vi "ReadWaveformFromFile.vi"() -> ()   [LabVIEW 2019]
panel:
  out "Laugh":bool caption="OK"
  in  "stop":bool
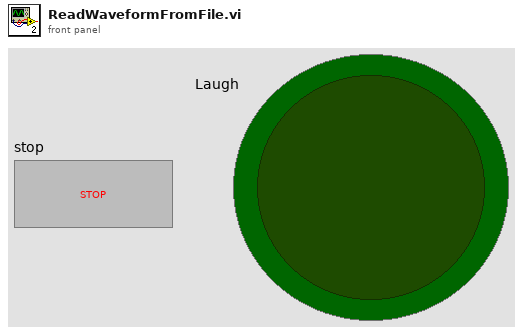
[diagram p1: front panel]
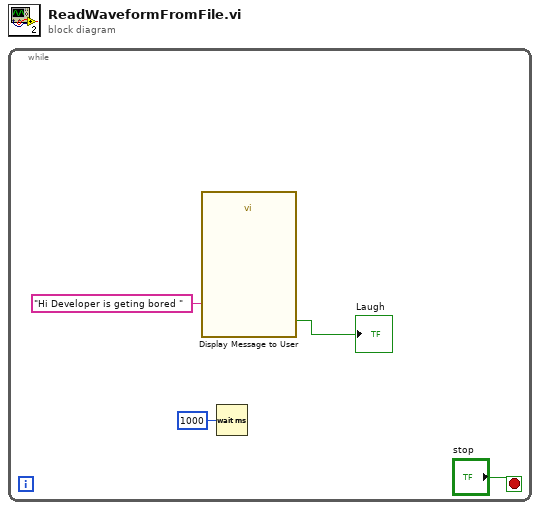
[diagram p0: block diagram]
diagram:
  n1 = while {
    stop <- "stop" stop-if-true
    n2 = call "Display Message to User"("Message"="Hi Developer is geting bored ") -> ("OK"=→"Laugh":bool)  [unwired: 9 in, 1 out]
    n3 = Wait (ms)(milliseconds to wait=u32 1000) -> ()  [unwired: 1 out]
  }
